vi "AlazarConfigureSampleSkipping.vi"(0 "Handle":u64, 5 "Mode":u32(ring) items=["Disable", "Enable"], 7 "Sample Clocks Per Record":u32, 9 "Sample Skip Bitmap":u16[](array[numeric]), 11 "error in (no error)":errorcluster) -> (4 "Handle":u64, 10 "Return Code":u32, 15 "error out":errorcluster)   [LabVIEW 2009]
doc: "Use this function to allow the digitizer to sub-sample post trigger data in arbitrary, non-uniform intervals. The application specifies which sample clock edges after a trigger event that the digitizer should use to generate sample points, and which sample clock edges that the digitizer should ignore."
uses:
  ATSApi.dll
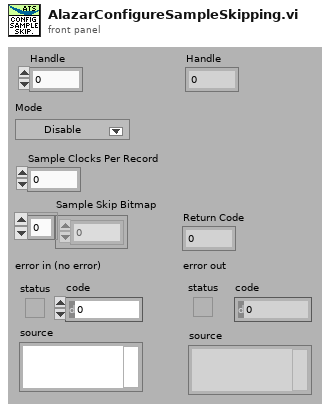
[diagram p1: front panel]
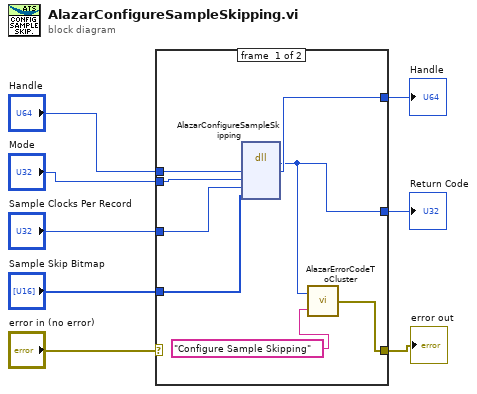
[diagram p0: block diagram]
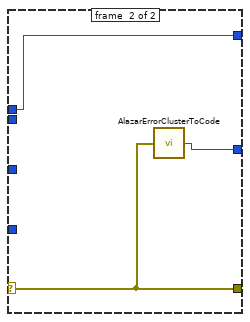
[diagram p2: hidden frame]
diagram:
  n1 = case shown="No Error" "error in (no error)" {
    selector: "error in (no error)" -> [_ w19]
    tunnel: [w10 w19] -> w7
    tunnel: "Handle" -> [w16 w18]
    tunnel: [w15 w18] -> w5
    tunnel: "Mode" -> [w14 _]
    tunnel: "Sample Clocks Per Record" -> [w13 _]
    tunnel: "Sample Skip Bitmap" -> [w12 _]
    tunnel: [w11 w17] -> w1
    frame #0 {
      n2 = dll-call lib="ATSApi.dll" fn="AlazarConfigureSampleSkipping"("handle"=w16, "Mode"=w14, "sampleClocksPerSecond"=w13, "pSampleSkipBitmap"=w12) -> ("return type"=w11:u32, "handle"=w15:u64)  [unwired: 6 in, 2 out]
      n3 = call "AlazarErrorCodeToCluster.vi"("Message"="Configure Sample Skipping", "Error Code"=w11) -> ("error out"=w10:errorcluster)
    }
    frame #1 {
      n4 = call "AlazarErrorClusterToCode.vi"("error in (no error)"=w19) -> ("Error Code"=w17:u32)
    }
  }
  "Handle" <- w5
  "error out" <- w7
  "Return Code" <- w1
